vi "Load Category Summaries.vi"(8 "error in (no error)":errorcluster, 10 "Year-Mo":string, 11 "Database in":refnum<class "Database.lvclass">) -> (0 "error out":errorcluster, 2 "Category Summaries":refnum<class "Expense Summary.lvclass">[](array[class]), 3 "Database out":refnum<class "Database.lvclass">)   [LabVIEW 2018, in "Database.lvclass"]
uses:
  Database.lvclass
  Expense Summary/Expense Summary.lvclass
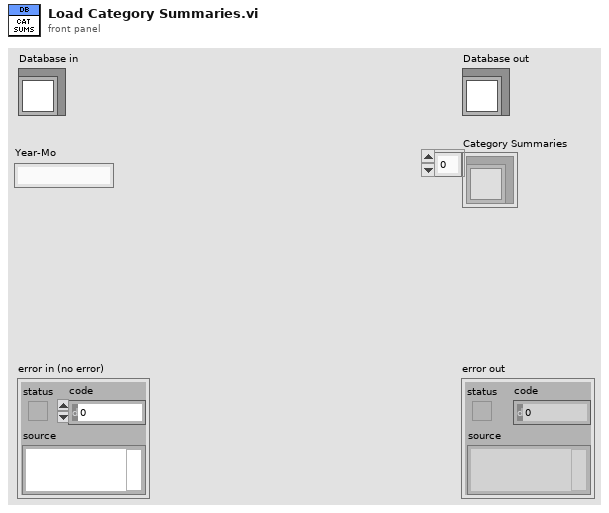
[diagram p1: front panel]
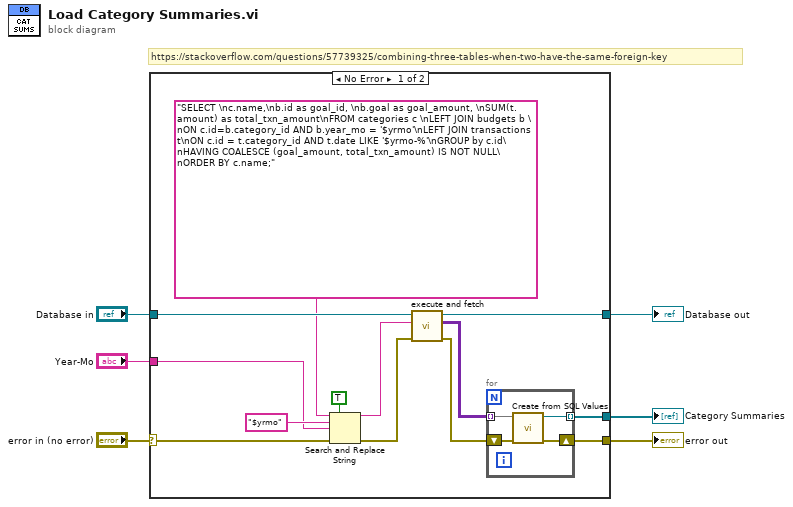
[diagram p0: block diagram]
diagram:
  # "https://stackoverflow.com/questions/57739325/combining-three-tables-when-two-have-the-same-foreign-key"
  n1 = case shown="No Error" "error in (no error)" {
    selector: "error in (no error)" -> [w14 w24]
    tunnel: [w17 w25] -> w6
    tunnel: "Database in" -> [w16 w25]
    tunnel: [w15 w24] -> w4
    tunnel: "Year-Mo" -> [w10 _]
    tunnel: [w7 _] -> w1
    frame No Error {
      n2 = Search and Replace String(replace all?=TRUE ("replace all? (F)"), input string="SELECT \nc.name,\nb.id as goal_id, \nb.goal as goal_amount, \nSUM(t.amount) as total_txn_amount\nFROM categories c \nLEFT JOIN budgets b \nON c.id=b.category_id AND b.year_mo = '$yrmo'\nLEFT JOIN transactions t\nON c.id = t.category_id AND t.date LIKE '$yrmo-%'\nGROUP by c.id\nHAVING COALESCE (goal_amount, total_txn_amount) IS NOT NULL\nORDER BY c.name;", search string="$yrmo", replace string=w10, error in=w14) -> (result string=w8:string, error out=w9:errorcluster)  [unwired: 3 in, 2 out]
      n3 = call "execute and fetch.vi"("error in (no error)"=w9, "SQL query"=w8, "Database in"=w16) -> ("error out"=w18:errorcluster, "recordset data"=w19:variant[][], "Database out"=w17:refnum<class "Database.lvclass">)  [unwired: 5 in, 1 out]
      n4 = for {
        tunnel: w19 -> [w22] mode=indexing
        shift-right: [w20] -> w15
        shift-left: w18 -> [w23]
        tunnel: [w21] -> w7 mode=indexing
        n5 = call "Create from SQL Values.vi"("error in (no error)"=w23, "recordset data"=w22) -> ("error out"=w20:errorcluster, "Expense Summary out"=w21:refnum<class "Expense Summary.lvclass">)  [unwired: 8 in]
      }
    }
    frame Error {
    }
  }
  "error out" <- w4
  "Database out" <- w6
  "Category Summaries" <- w1
